vi "Initialise.vi"(8 "error in (no error)":errorcluster, 10 "Message in":refnum<class "InitialiseMessage.lvclass">, 11 "focus in":refnum<class "focus.lvclass">) -> (0 "error out":errorcluster, 3 "focus out":refnum<class "focus.lvclass">)   [LabVIEW 2012, in "focus.lvclass"]
doc: "This method is called when an initialise message is received. It mainly initialises the RabbitMQ connectivity. \n\nOverride this method when your component needs special initialisation (e.g. of software or hardware resources). In that case, don't forget to call the parent for proper implementation. If your component owns subcomponents, they count as resources, so you have to initialise them by calling their own initialise functions"
uses:
  focus.lvclass
  <vilib>/Distrio/Murmex/InitialiseMessage/InitialiseMessage.lvclass
  <vilib>/Distrio/Murmex/Murmex/Murmex.lvclass
  focus.lvclass/focus.ctl
panel:
  # "This method is called when the INTIALISE\ntrigger is sent. \n\nOverride this method when your component needs to\nrespond to this trigger. \n\nCall parent for proper implementation"
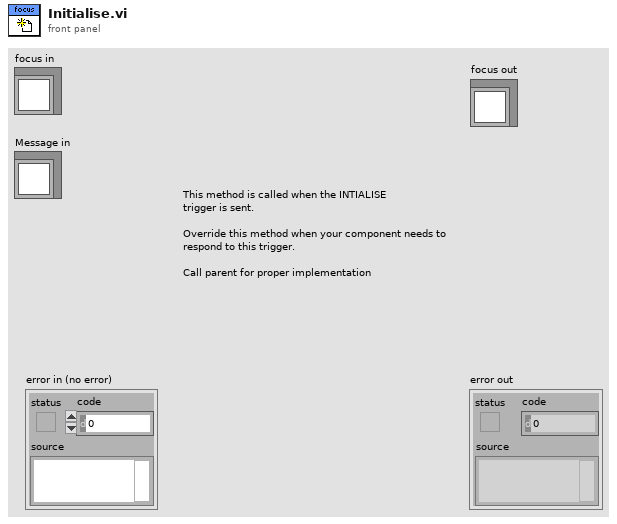
[diagram p1: front panel]
types:
  T1 = cluster{"Register DC":bool, "DaisyChain Search?":bool, "Device ID":i32}[][]
  T2 = cluster{"RON Affected axes":string[], "Reference mode":bool[], "Check FRF?":bool}
  T3 = typedef "focus.lvclass/port_focus.ctl" = i32
  T4 = typedef "focus.lvclass/baud_rate_focus.ctl" = u16
  T5 = typedef "focus.lvclass/connection_type_focus.ctl" = enum16{"RS232", "RS232 DaisyChain", "USB", "USB_DaisyChain"}
  T6 = cluster{"Register DC":bool, "DaisyChain Search?":bool, "Device ID":i32}
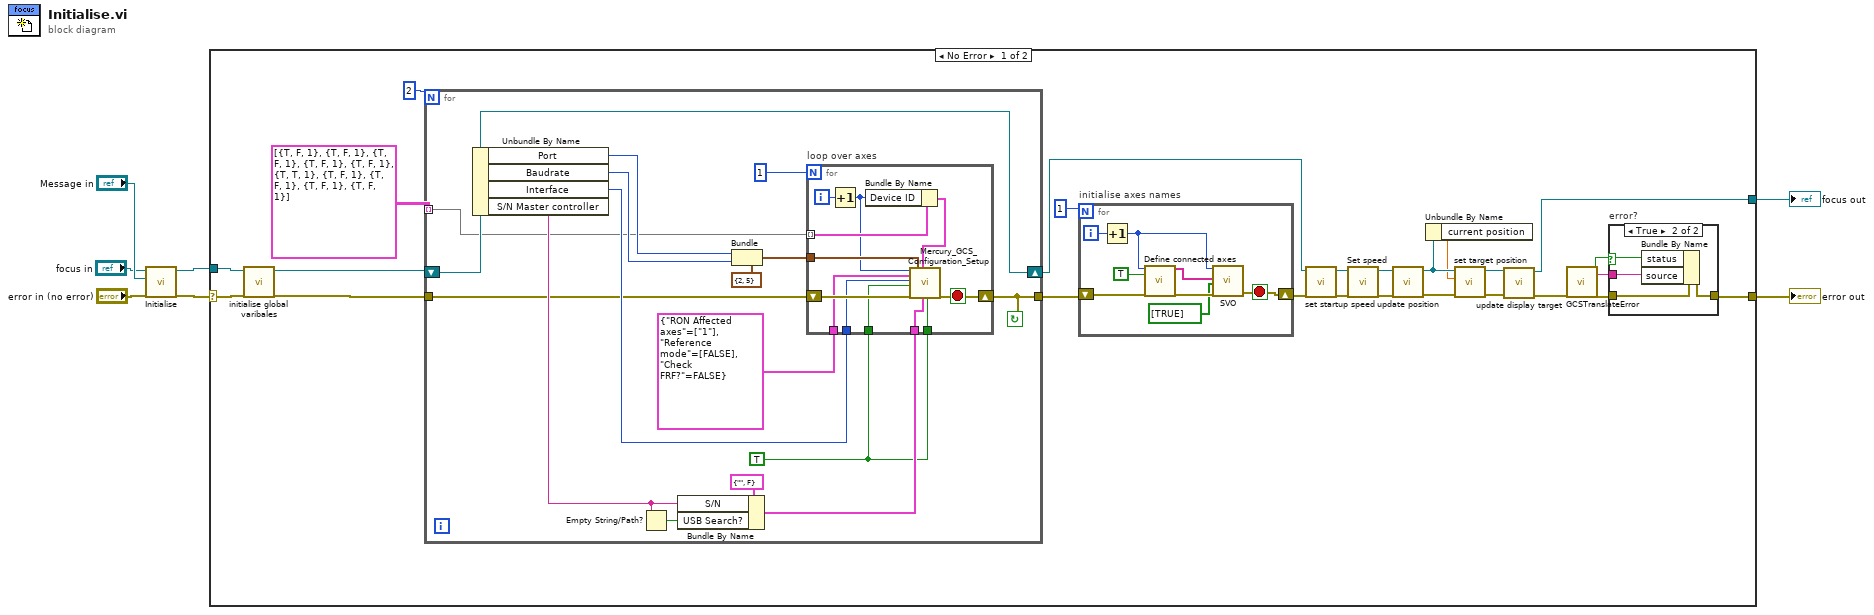
[diagram p0: block diagram]
diagram:
  n1 = call-parent "Initialise.vi"("error in (no error)"="error in (no error)", "Message in"="Message in", "Murmex in"="focus in") -> ("error out"=w4:errorcluster, "Murmex out"=w3:refnum<class "focus.lvclass">)  [unwired: 7 in]
  n2 = case shown="No Error" w4 {
    selector: w4 -> [w31 w74]
    tunnel: w3 -> [w32 w75]
    tunnel: [w23 w74] -> w1
    tunnel: [w9 w75] -> w2
    frame No Error {
      n3 = call-dynamic "initialise global varibales.vi"("error in (no error)"=w31, "focus in"=w32) -> ("error out"=w30:errorcluster, "focus out"=w29:refnum<class "focus.lvclass">)  [unwired: 8 in]
      n4 = for {
        N: 2 -> [_]
        tunnel: w30 -> [w50]
        shift-right: [w55] -> w10
        shift-left: w29 -> [w55]
        tunnel: [w49] -> w25
        tunnel: T1 [[{"Register DC"=TRUE, "DaisyChain Search?"=FALSE, "Device ID"=1}, {"Register DC"=TRUE, "DaisyChain Search?"=FALSE, "Device ID"=1}, {"Register DC"=TRUE, "DaisyChain Search?"=FALSE, "Device ID"=1}, {"Register DC"=TRUE, "DaisyChain Search?"=FALSE, "Device ID"=1}, {"Register DC"=TRUE, "DaisyChain Search?"=FALSE, "Device ID"=1}], [{"Register DC"=TRUE, "DaisyChain Search?"=TRUE, "Device ID"=1}, {"Register DC"=TRUE, "DaisyChain Search?"=FALSE, "Device ID"=1}, {"Register DC"=TRUE, "DaisyChain Search?"=FALSE, "Device ID"=1}, {"Register DC"=TRUE, "DaisyChain Search?"=FALSE, "Device ID"=1}, {"Register DC"=TRUE, "DaisyChain Search?"=FALSE, "Device ID"=1}]] -> [w47] mode=indexing
        stop <- w49 continue-if-true
        w51 = TRUE ("Switch servo on?")
        n5 = Unbundle By Name(w55) -> ("Port"=w57:T3, "Baudrate"=w56:T4, "Interface"=w53:T5, "S/N Master controller"=w59:string)
        n6 = Empty String/Path?(string/path=w59) -> (empty?=w60:bool)
        n7 = Bundle By Name(cluster=cluster{"S/N":string, "USB Search?":bool} {"S/N"="", "USB Search?"=FALSE} ("USB settings"), "S/N"=w59, "USB Search?"=w60) -> (w52:cluster{"S/N":string, "USB Search?":bool})
        n8 = Bundle(cluster=cluster{"Portnumber":i32, "Baudrate":u16} {"Portnumber"=2, "Baudrate"=5} ("RS232 settings"), "Portnumber"=w57, "Baudrate"=w56) -> (w48:cluster{"Portnumber":i32, "Baudrate":u16})
        n9 = for "loop over axes" {
          N: 1 -> [_]
          tunnel: T2 {"RON Affected axes"=["1"], "Reference mode"=[FALSE], "Check FRF?"=FALSE} ("RON settings") -> [w67]
          tunnel: w53 -> [w66]
          tunnel: w51 -> [w65]
          tunnel: w52 -> [w63]
          tunnel: w51 -> [w64]
          shift-right: [w62] -> w49
          shift-left: w50 -> [w73]
          tunnel: w48 -> [w72]
          tunnel: w47 -> [w70] mode=indexing
          i -> [w71]
          stop <- w62 stop-if-true
          n10 = Increment(x=w71) -> (x+1=w68:i32)
          n11 = Bundle By Name(cluster=w70, "Device ID"=w68) -> (w69:T6)
          n12 = call "Mercury_GCS_Configuration_Setup.vi"("System no."=w68, "RON settings"=w67, "Interface"=w66, "All axes?"=w65, "error in"=w73, "RS232 settings"=w72, "DaisyChain settings"=w69, "USB settings"=w63, "Switch servo on?"=w64) -> ("error out"=w62:errorcluster)  [unwired: 4 in, 6 out]
        }
      }
      n13 = for "initialise axes names" {
        N: 1 -> [_]
        shift-right: [w38] -> w20
        shift-left: w25 -> [w43]
        i -> [w45]
        stop <- w38 stop-if-true
        n14 = Increment(x=w45) -> (x+1=w39:i32)
        n15 = call "Define connected axes.vi"("System no."=w39, "Read from\ncontroller?"=TRUE ("Read from\ncontroller?"), "error in"=w43) -> ("Conn. Axes out"=w41:string[], "error out"=w42:errorcluster)  [unwired: 15 in]
        n16 = call "SVO.vi"("System no."=w39, "Axes to command"=w41, "Servo mode"=bool[] [TRUE], "error in"=w42) -> ("error out"=w38:errorcluster)  [unwired: 15 in]
      }
      n17 = call-dynamic "set startup speed.vi"("error in (no error)"=w20, "focus in"=w10) -> ("error out"=w19:errorcluster, "focus out"=w18:refnum<class "focus.lvclass">)  [unwired: 8 in]
      n18 = call-dynamic "Set speed.vi"("error in (no error)"=w19, "focus in"=w18) -> ("error out"=w17:errorcluster, "focus out"=w16:refnum<class "focus.lvclass">)  [unwired: 8 in]
      n19 = call-dynamic "update position.vi"("error in (no error)"=w17, "focus in"=w16) -> ("error out"=w14:errorcluster, "focus out"=w15:refnum<class "focus.lvclass">)  [unwired: 8 in]
      n20 = Unbundle By Name(w15) -> ("current position"=w8:dbl)
      n21 = call-dynamic "set target position.vi"("error in (no error)"=w14, "target position"=w8, "focus in"=w15) -> ("error out"=w13:errorcluster, "focus out"=w12:refnum<class "focus.lvclass">)  [unwired: 7 in]
      n22 = call-dynamic "update display target.vi"("error in (no error)"=w13, "focus in"=w12) -> ("error out"=w11:errorcluster, "focus out"=w9:refnum<class "focus.lvclass">)  [unwired: 8 in]
      n23 = call "GCSTranslateError.vi"("error in"=w11) -> ("GCS Error?"=w22:bool, "Error Description"=w21:string, "error out"=w24:errorcluster)  [unwired: 16 in]
      n24 = case "error?" shown="True" w22 {
        selector: w22 -> [_ w36]
        tunnel: w24 -> [w33 w37]
        tunnel: [w33 w35] -> w23
        tunnel: w21 -> [_ w34]
        frame False {
        }
        frame True {
          n25 = Bundle By Name(cluster=w37, "status"=w36, "source"=w34) -> (w35:errorcluster)
        }
      }
    }
    frame Error {
    }
  }
  "error out" <- w1
  "focus out" <- w2
